vi "Network Command Engine.vi"(8 "error in (no error)":errorcluster, 11 "State Variables":T1) -> (0 "error out":errorcluster)   [LabVIEW 2015, in "Instrument Addon Engine.lvlib" / "Network Common API.lvlib"]
uses:
  Network Common API.lvlib
  Types/Engine State Variables.ctl
  <vilib>/NI/NI VeriStand Inline Async API/_VS Inline Async API/Process/Process.lvclass
  TCP Refs.ctl
  Network Comm Global Ref.ctl
  <vilib>/NI/AMC/Message Queue.ctl
  <vilib>/NI/AMC/Message.ctl
  <vilib>/NI/Tools/Keyed Array/KeyedArray.ctl
  <vilib>/NI/NI VeriStand Inline Async API/_Data Access Engine/Access Type Classes/Write/Write.lvclass
  <vilib>/NI/NI VeriStand Inline Async API/_Data Access Engine/Access Type Classes/Read/Read.lvclass
  <vilib>/NI/NI VeriStand Inline Async API/_Data Access Engine/Access Type Classes/ReadWrite/ReadWrite.lvclass
  <vilib>/NI/STM/compatibility/stm_TCPConnectionMethod.ctl
  <vilib>/NI/STM/compatibility/stm_TCP Read Options.ctl
  <vilib>/NI/NI VeriStand Inline Async API/_VS Inline Async API/Process/Process.lvclass/Process.ctl
  <vilib>/NI/AMC/Create Single Message.vi
  <vilib>/NI/AMC/Update Message Routing Info.vi
  <vilib>/NI/Tools/Keyed Array/Map String.vi
  <vilib>/NI/AMC/Read Termination Message.vi
  <vilib>/NI/NI VeriStand Inline Async API/_VS Inline Async API/Error Handling Process/SubVIs/Error.ConvertArray.vi
  <vilib>/NI/Tools/String/Get Case Matching.vi
  <vilib>/NI/STM/compatibility/STM Get Connection Reference (TCP).vi
  <vilib>/NI Veristand/Custom Device Tools/Custom Device Utility Library/NI VeriStand - Print Debug String.vi
  <vilib>/NI/STM/compatibility/STM Write Message (TCP).vi
  <vilib>/NI/AMC/Globals.vi
  <vilib>/NI/AMC/Send Message.vi
  Shared/Constants.vi
  <vilib>/NI/STM/compatibility/STM Read Message (TCP).vi
  <vilib>/NI/AMC/AMC.lvlib
  <vilib>/NI/Tools/Keyed Array/Tools_KeyedArray.lvlib
  Shared/Instrument Addon Shared.lvlib
  Instrument Addon Engine.lvlib
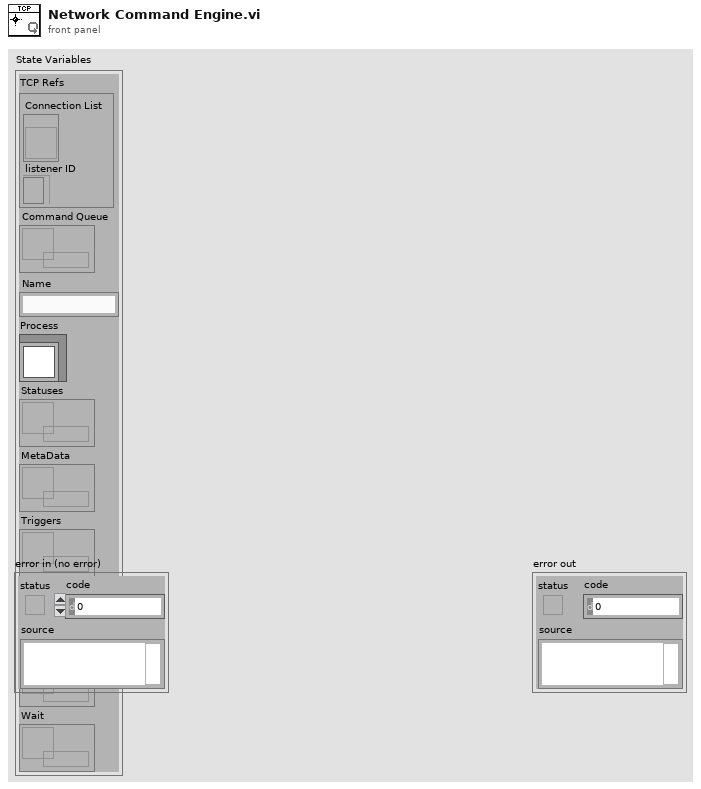
[diagram p1: front panel]
types:
  T1 = typedef "Instrument Addon Engine.lvlib/Engine State Variables.ctl" = cluster{"TCP Refs":T2, "Command Queue":T4, "Name":string, "Process":refnum<class "Process.lvclass">, "Statuses":refnum<data-value>, "MetaData":refnum<data-value>, "Triggers":refnum<data-value>, "Periodic Enable":refnum<data-value>, "Data":refnum<data-value>, "Wait":refnum<data-value>}
  T2 = typedef "Instrument Addon Engine.lvlib/Network Common API.lvlib/TCP Refs.ctl" = cluster{"Connection List":T3, "listener ID":refnum<k5>}
  T3 = typedef "Instrument Addon Engine.lvlib/Network Common API.lvlib/Network Comm Global Ref.ctl" = refnum<vi>
  T4 = typedef "AMC.lvlib/Message Queue.ctl" = refnum<queue>
  T5 = typedef "stm_TCPConnectionMethod.ctl" = enum16{"Initialize", "Add Connection", "Set Properties", "Get Connection(s)", "Remove Connection", "Remove All Connections", "Get Connection Count"}
  T6 = typedef "stm_TCP Connection Info.ctl" = cluster{"connection ID":refnum<k5>, "Meta data":T7[]}
  T7 = typedef "stm_MetaDataElement.ctl" = string
  T8 = typedef "stm_TCP Read Options.ctl" = cluster{"Ignore Timeout Error":bool, "timeout ms (1000)":i32}
  T9 = typedef "Tools_KeyedArray.lvlib/KeyedArray.ctl" = cluster{"keys":string[], "values":string[]}
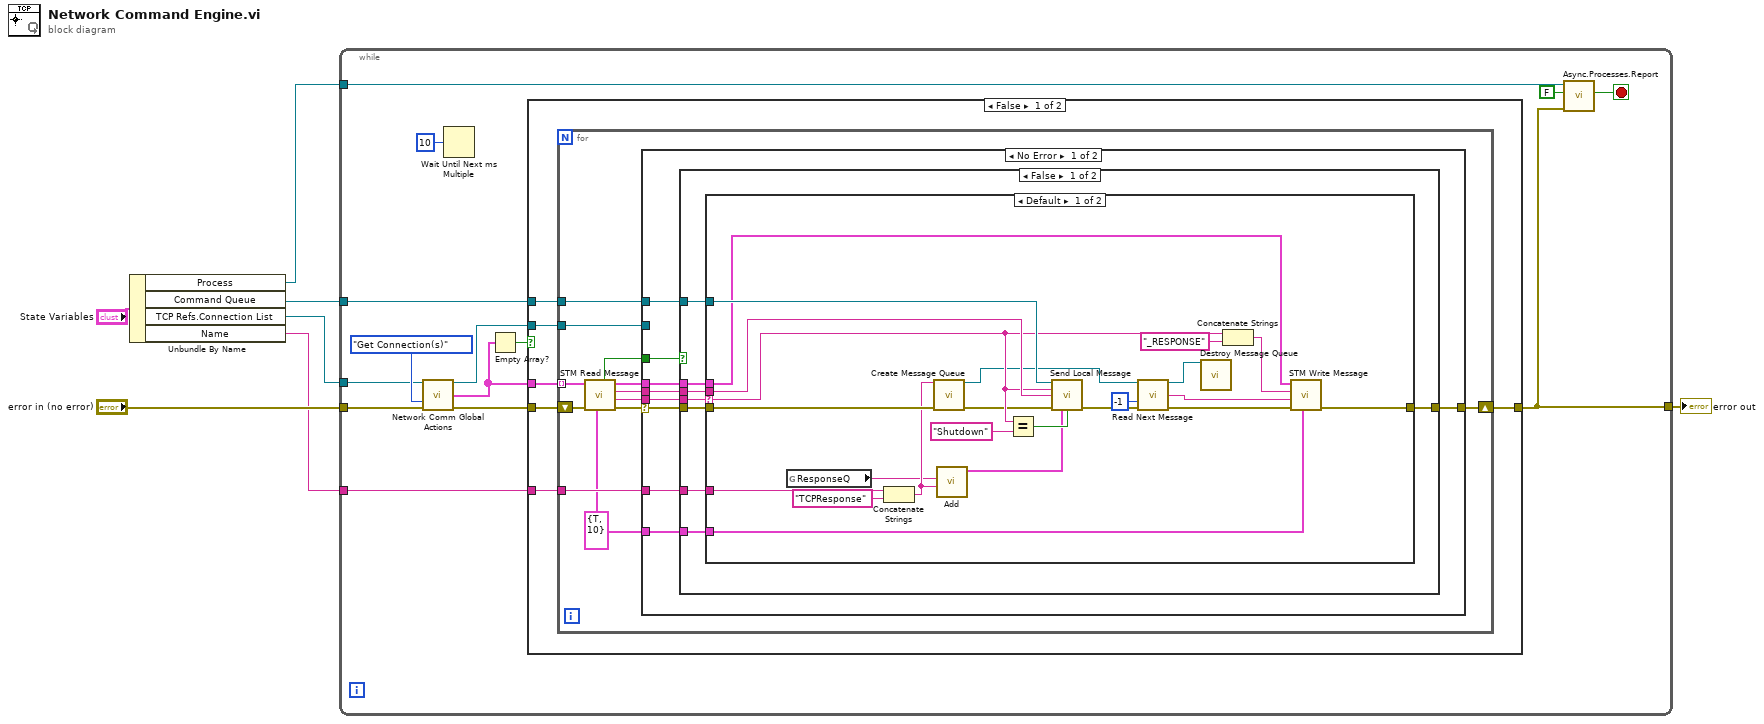
[diagram p0: block diagram]
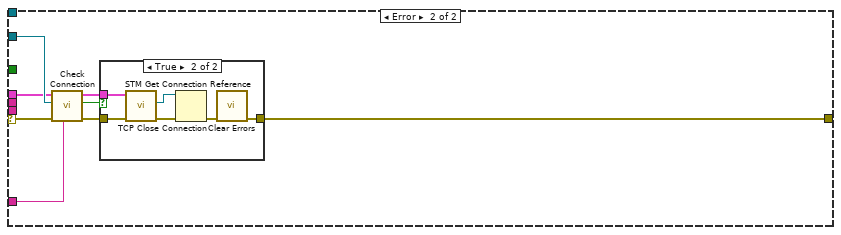
[diagram p4: hidden frame]
diagram:
  n1 = Unbundle By Name("State Variables") -> ("Process"=w7:refnum<class "Process.lvclass">, "Command Queue"=w1:T4, "TCP Refs.Connection List"=w5:T3, "Name"=w2:string)
  n2 = while {
    tunnel: "error in (no error)" -> [w17]
    tunnel: [w8] -> w3
    tunnel: w5 -> [w13]
    tunnel: w7 -> [w12]
    tunnel: w2 -> [w11]
    tunnel: w1 -> [w9]
    stop <- w14 stop-if-true
    n3 = call "Network Comm Global Actions.vi"("ref in"=w13, "Method"=stm_TCPConnectionMethod."Get Connection(s)", "error in (no error)"=w17) -> ("ref out"=w15:T3, "All Connections"=w18:T6[], "error out"=w16:errorcluster)  [unwired: 6 in, 4 out]
    n4 = Wait Until Next ms Multiple(millisecond multiple=u32 10 ("STM Update Rate")) -> ()  [unwired: 1 out]
    n5 = Empty Array?(array=w18) -> (empty?=w19:bool)
    n6 = case shown="False" w19 {
      tunnel: w18 -> [w27 _]
      tunnel: w16 -> [w23 w97]
      tunnel: w15 -> [w26 _]
      tunnel: [w25 w97] -> w8
      tunnel: w11 -> [w24 _]
      tunnel: w9 -> [w22 _]
      frame False {
        n7 = for {
          tunnel: w27 -> [w34] mode=indexing
          tunnel: w26 -> [w39]
          shift-right: [w38] -> w25
          shift-left: w23 -> [w36]
          tunnel: w24 -> [w37]
          tunnel: w22 -> [w29]
          w28 = T8 {"Ignore Timeout Error"=TRUE, "timeout ms (1000)"=10} ("options")
          n8 = call-poly <vilib>:"STM Read Message.vi"("Options"=w28, "error in"=w36, "Connection Info"=w34) -> ("error out"=w35:errorcluster, "Name"=w31:T7, "data string"=w32:string, "Connection Info Out"=w33:T6, "Timed Out?"=w30:bool)  [unwired: 3 in, 1 out]
          n9 = case shown="No Error" w35 {
            selector: w35 -> [w48 w84]
            tunnel: w39 -> [_ w86]
            tunnel: w33 -> [w42 w85]
            tunnel: [w47 w83] -> w38
            tunnel: w37 -> [w41 w82]
            tunnel: w32 -> [w46 _]
            tunnel: w31 -> [w45 _]
            tunnel: w30 -> [w44 _]
            tunnel: w29 -> [w43 _]
            tunnel: w28 -> [w40 _]
            frame No Error {
              n10 = case shown="False" w44 {
                tunnel: w48 -> [w53 w81]
                tunnel: [w56 w81] -> w47
                tunnel: w46 -> [w51 _]
                tunnel: w45 -> [w52 _]
                tunnel: w43 -> [w55 _]
                tunnel: w42 -> [w54 _]
                tunnel: w41 -> [w50 _]
                tunnel: w40 -> [w49 _]
                frame False {
                  n11 = case shown="Default" w52 {
                    selector: w52 -> [w70 _]
                    tunnel: w53 -> [w79 w80]
                    tunnel: [w74 w80] -> w56
                    tunnel: w51 -> [w78 _]
                    tunnel: w55 -> [w76 _]
                    tunnel: w54 -> [w73 _]
                    tunnel: w50 -> [w77 _]
                    tunnel: w49 -> [w68 _]
                    frame Default {
                      n12 = global read "Constants.vi" "ResponseQ"() -> (w57:string)
                      n13 = Concatenate Strings(w77, "TCPResponse" ("message name")) -> (w62:string)
                      n14 = call <vilib>:"Create Message Queue.vi"("message queue name"=w62, "error in"=w79) -> ("message queue out"=w60:T4, "error out"=w65:errorcluster)  [unwired: 12 in]
                      n15 = call <vilib>:"Add.vi"("value"=w62, "key"=w57) -> ("array out"=w63:T9)  [unwired: 3 in, 2 out]
                      n16 = Equal?(x=w70, y="Shutdown" ("x")) -> (x = y?=w67:bool)
                      n17 = call <vilib>:"Send Local Message.vi"("message queue in"=w76, "message name"=w70, "message value"=w78, "error in"=w65, "message attributes"=w63, "priority message (F)"=w67) -> ("error out"=w61:errorcluster)  [unwired: 7 in, 2 out]
                      n18 = call <vilib>:"Read Next Message.vi"("message queue in"=w60, "timeout (1 ms)"=-1, "error in"=w61) -> ("message queue out"=w58:T4, "message value"=w72:string, "error out"=w75:errorcluster)  [unwired: 5 in, 5 out]
                      n19 = call <vilib>:"Destroy Message Queue.vi"("message queue in"=w58) -> ()  [unwired: 12 in, 3 out]
                      n20 = Concatenate Strings(w70, "_RESPONSE" ("string")) -> (w69:string)
                      n21 = call-poly <vilib>:"STM Write Message.vi"("Options"=w68, "error in (no error)"=w75, "Data"=w72, "Name"=w69, "Connection Info"=w73) -> ("error out"=w74:errorcluster)  [unwired: 5 in, 1 out]
                    }
                    frame "" {
                    }
                  }
                }
                frame True {
                }
              }
            }
            frame Error {
              n22 = call "Check Connection.vi"("Name"=w82, "error in (no error)"=w84, "ref in"=w86, "Connection In"=w85) -> ("error out"=w89:errorcluster, "Disconnected"=w87:bool, "Connection In"=w88:T6)  [unwired: 5 in]
              n23 = case shown="True" w87 {
                tunnel: [w90 w93] -> w83
                tunnel: w89 -> [w90 w96]
                tunnel: w88 -> [_ w91]
                frame False {
                }
                frame True {
                  n24 = call-poly <vilib>:"STM Get Connection Reference.vi"("error in"=w96, "Connection Info"=w91) -> ("error out"=w95:errorcluster, "connection ID out"=w94:refnum<k5>)  [unwired: 7 in, 1 out]
                  n25 = TCP Close Connection(connection ID=w94, error in (no error)=w95) -> (error out=w92:errorcluster)  [unwired: 1 in, 1 out]
                  n26 = call <vilib>:"Clear Errors.vi"("error in (no error)"=w92) -> ("error out"=w93:errorcluster)  [unwired: 5 in, 1 out]
                }
              }
            }
          }
        }
      }
      frame True {
      }
    }
    n27 = call <vilib>:"Async.Processes.Report.vi"("Error"=w8, "Stop on Error?"=FALSE, "Process in"=w12) -> ("Stop"=w14:bool)  [unwired: 7 in, 1 out]
  }
  "error out" <- w3
